vi "AddToGroup Value Change.vi"(11 "References":T1) -> (0 "error out":errorcluster)   [LabVIEW 2015, in "TDMS datalogger editor node.lvclass"]
uses:
  TDMS datalogger editor node.lvclass
  <vilib>/NI/DCAF/Tag Editor Core/Table API/Table Manager/object ref.ctl
  <vilib>/NI/DCAF/Tag Editor Core/Configuration Editor/Classes/Engine Parent/Engine Parent Editor Node.lvclass
  <vilib>/NI/DCAF/Tag Editor Core/Configuration Editor/Classes/Module editor node/module editor node.lvclass
  TDMS datalogger editor node.lvclass/TDMS datalogger editor node.ctl
  <vilib>/NI/Tag Bus/tag/tag descriptor.lvclass/tag descriptor.ctl
  <vilib>/NI/Tag Bus/tag/tag descriptor.lvclass
  module/configuration/TDMS datalogger configuration.lvclass
  <vilib>/NI/DCAF/Tag Editor Core/Table API/Table Manager/Table Manager.lvclass
panel:
  in  "Groups":string(tree)="group1"
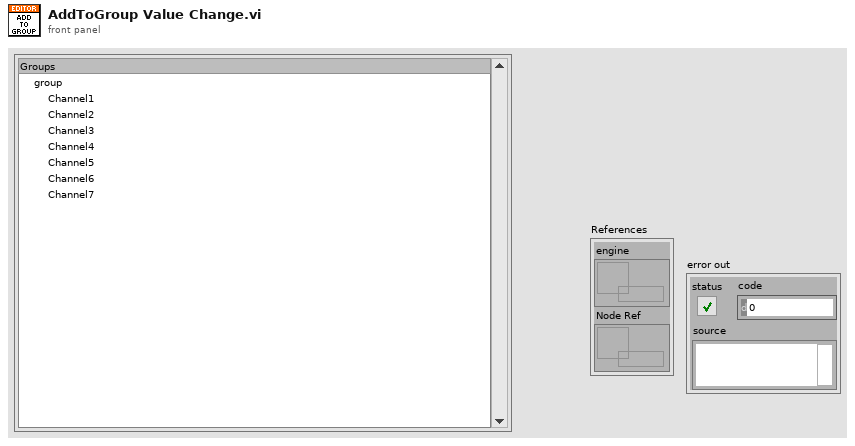
[diagram p1: front panel]
types:
  T1 = typedef "Table Manager.lvlib/Table Manager.lvclass/object ref.ctl" = cluster{"engine":refnum<data-value>, "Node Ref":refnum<data-value>}
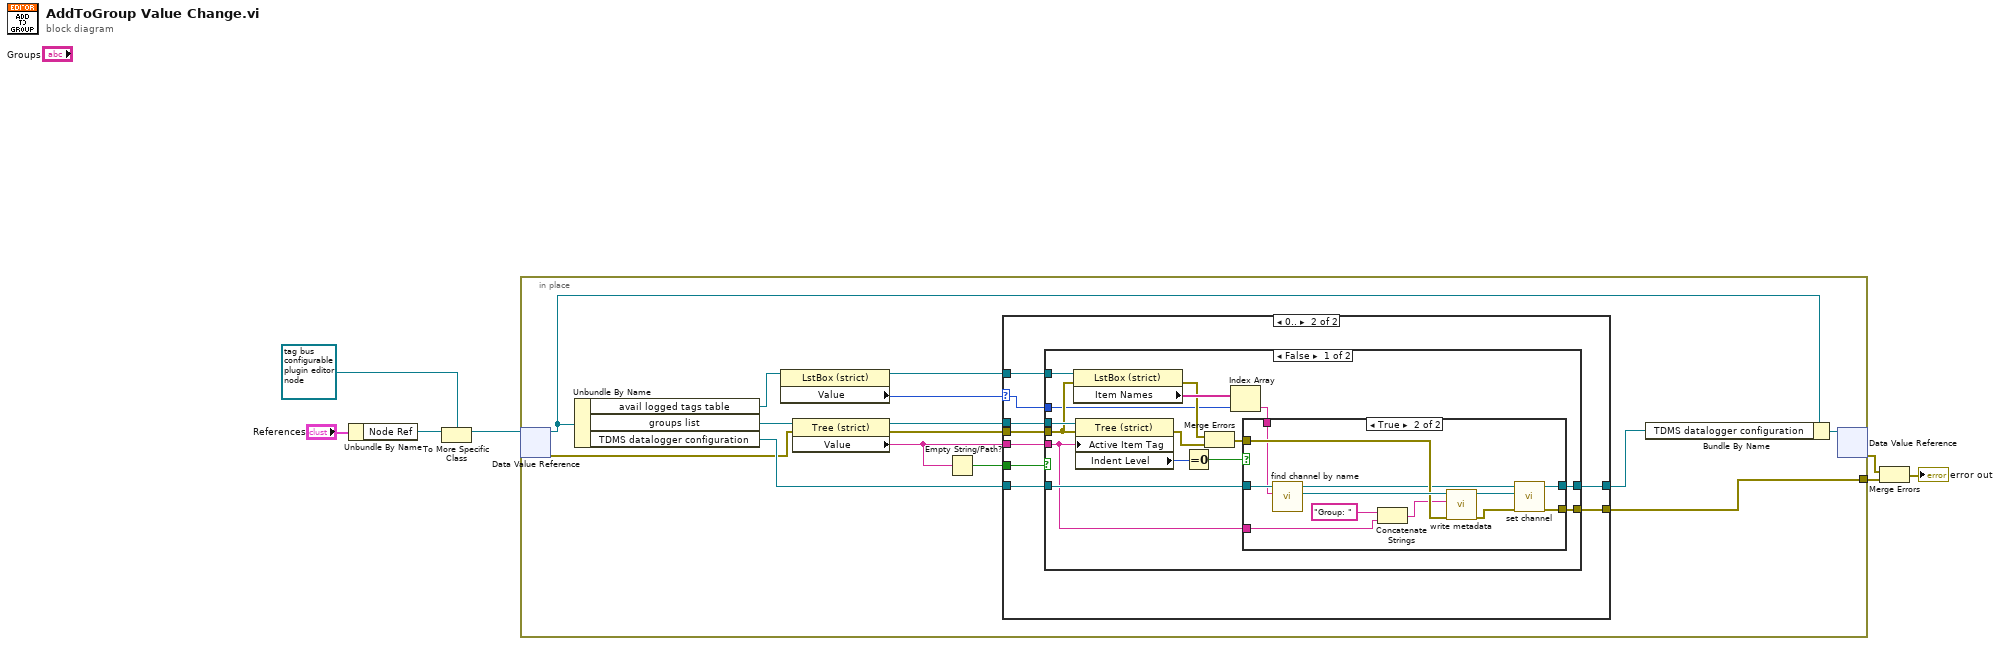
[diagram p0: block diagram]
diagram:
  n1 = Unbundle By Name("References") -> ("Node Ref"=w6:refnum<data-value>)
  n2 = To More Specific Class(target class=refnum<data-value> refnum ("data value reference"), reference=w6) -> (specific class reference=w4:refnum<data-value>)  [unwired: 1 in, 1 out]
  n3 = in-place {
    in-place-border: [w21] -> w3
    n4 = in-place-dvr #1(w4) -> (w19:refnum<class "TDMS datalogger editor node.lvclass">, w10:errorcluster)
    n5 = Unbundle By Name(w19) -> ("avail logged tags table"=w15:refnum<vi>, "groups list"=w12:refnum<vi>, "TDMS datalogger configuration"=w20:refnum<class "TDMS datalogger configuration.lvclass">)
    n6 = property class="LstBox (strict)"(reference=w15) -> (reference out=w14:refnum<vi>, "Value"=w13:i32)  [unwired: 1 in, 1 out]
    n7 = property class="Tree (strict)"(reference=w12, error in=w10) -> (reference out=w11:refnum<vi>, error out=w9:errorcluster, "Value"=w8:string)
    n8 = Empty String/Path?(string/path=w8) -> (empty?=w16:bool)
    n9 = case shown="0.." w13 {
      selector: w13 -> [_ w24]
      tunnel: [w22 w32] -> w21
      tunnel: w11 -> [_ w31]
      tunnel: w20 -> [w23 w30]
      tunnel: w9 -> [w22 w29]
      tunnel: [w23 w28] -> w17
      tunnel: w16 -> [_ w27]
      tunnel: w8 -> [_ w26]
      tunnel: w14 -> [_ w25]
      frame ..-1 {
        # "Do Nothing if no Channel selected"
      }
      frame 0.. {
        n10 = case shown="False" w27 {
          tunnel: [w47 w62] -> w32
          tunnel: w31 -> [w46 _]
          tunnel: w30 -> [w45 w63]
          tunnel: w25 -> [w41 _]
          tunnel: w29 -> [w38 w62]
          tunnel: w26 -> [w35 _]
          tunnel: [w34 w63] -> w28
          tunnel: w24 -> [w33 _]
          frame False {
            n11 = property class="LstBox (strict)"(reference=w41, error in=w38) -> (error out=w36:errorcluster, "Item Names"=w40:string[])  [unwired: 1 out]
            n12 = property class="Tree (strict)"(reference=w46, error in=w38, "Active Item Tag"=w35) -> (error out=w44:errorcluster, "Indent Level"=w43:i32)  [unwired: 1 out]
            n13 = Equal To 0?(x=w43) -> (x = 0?=w42:bool)
            n14 = Merge Errors(w36, w44) -> (w37:errorcluster)
            n15 = Index Array(array=w40, index=w33) -> (element=w39:string)
            n16 = case shown="True" w42 {
              tunnel: [w49 w53] -> w47
              tunnel: w45 -> [w48 w61]
              tunnel: w35 -> [_ w56]
              tunnel: w37 -> [w49 w59]
              tunnel: w39 -> [_ w58]
              tunnel: [w48 w51] -> w34
              frame False {
                # "Don't add to channel items"
              }
              frame True {
                n17 = call "find channel by name.vi"("channel name"=w58, "TDMS datalogger configuration in"=w61) -> ("channel"=w60:refnum<class "TBM channel.lvclass">, "TDMS datalogger configuration out"=w52:refnum<class "TDMS datalogger configuration.lvclass">)  [unwired: 8 in]
                n18 = Concatenate Strings("Group: " ("string"), w56) -> (w55:string)
                n19 = call <vilib>:"write metadata.vi"("error in"=w59, "metadata"=w55, "system tag in"=w60) -> ("error out"=w54:errorcluster, "system tag out"=w50:refnum<class "TBM channel.lvclass">)  [unwired: 7 in]
                n20 = call "set channel.vi"("error in"=w54, "TBM channel in"=w50, "TDMS datalogger configuration in"=w52) -> ("error out"=w53:errorcluster, "TDMS datalogger configuration out"=w51:refnum<class "TDMS datalogger configuration.lvclass">)  [unwired: 7 in]
              }
            }
          }
          frame True {
            # "Do nothing if no group item selected"
          }
        }
      }
    }
    n21 = Bundle By Name(cluster=w19, "TDMS datalogger configuration"=w17) -> (w18:refnum<class "TDMS datalogger editor node.lvclass">)
    n22 = in-place-dvr #1(w18) -> (w2:errorcluster)  [unwired: 1 out]
  }
  n23 = Merge Errors(w2, w3) -> (→"error out":errorcluster)
